vi "ZLIB Write File__ogtk.vi"(5 "error in (no error)":errorcluster, 7 "source path":path, 8 "zip Refnum":T1) -> (0 "error out":errorcluster, 3 "zip Refnum out":T1)   [LabVIEW 2014]
doc: "Writes a file from disk into the ZIP archive at the currently created file entry."
uses:
  <userlib>/_OpenG.lib/lvzip/lvzip.llb/ZLIB Zip Handle__ogtk.ctl
  <userlib>/_OpenG.lib/lvzip/lvzlib.dll
panel:
  # "Please visit http://www.OpenG.org to learn about the\nOpen Source LabVIEW software movement.\n\nNOTICE -- YOU MUST LEAVE THIS NOTICE IN PLACE.  PER THE TERMS OF THE LICENSE BELOW, YOU MAY SUBLICENSE THIS SOFTWARE \nIN ANY WAY THAT DOES NOT CONFLICT WITH THIS LICENSE.\n\n### BSD License (http://www.opensource.org/licenses/bsd-license.php) Begin ###\n \nCopyright (C) 2002-2004 Rolf Kalbermatter rolf.kalbermatter@citeng.com\nCopyright (C) 2002 Jim Kring jim@jimkring.com\n\nAll rights reserved.\n\nRedistribution and use in source and binary forms, with or without modification, are permitted provided that the following conditions are met:\n\n    * Redistributions of source code must retain the above copyright notice, this list of conditions and the following disclaimer.\n    * Redistributions in binary form must reproduce the above copyright notice, this list of conditions and the following disclaimer in the \n       documentation and/or other materials provided with the distribution.\n    * Neither the name of SciWare, James Kring, Inc., nor the names of its contributors may be used to endorse or promote products derived \n       from this software without specific prior written permission.\n\nTHIS SOFTWARE IS PROVIDED BY THE COPYRIGHT HOLDERS AND CONTRIBUTORS \"AS IS\" AND ANY EXPRESS OR IMPLIED WARRANTIES, \nINCLUDING, BUT NOT LIMITED TO, THE IMPLIED WARRANTIES OF MERCHANTABILITY AND FITNESS FOR A PARTICULAR PURPOSE ARE \nDISCLAIMED. IN NO EVENT SHALL THE COPYRIGHT OWNER OR CONTRIBUTORS BE LIABLE FOR ANY DIRECT, INDIRECT, INCIDENTAL,\n SPECIAL, EXEMPLARY, OR CONSEQUENTIAL DAMAGES (INCLUDING, BUT NOT LIMITED TO, PROCUREMENT OF SUBSTITUTE GOODS OR \nSERVICES; LOSS OF USE, DATA, OR PROFITS; OR BUSINESS INTERRUPTION) HOWEVER CAUSED AND ON ANY THEORY OF LIABILITY, \nWHETHER IN CONTRACT, STRICT LIABILITY, OR TORT (INCLUDING NEGLIGENCE OR OTHERWISE) ARISING IN ANY WAY OUT OF THE USE \nOF THIS SOFTWARE, EVEN IF ADVISED OF THE POSSIBILITY OF SUCH DAMAGE.\n\n### BSD License End ###"
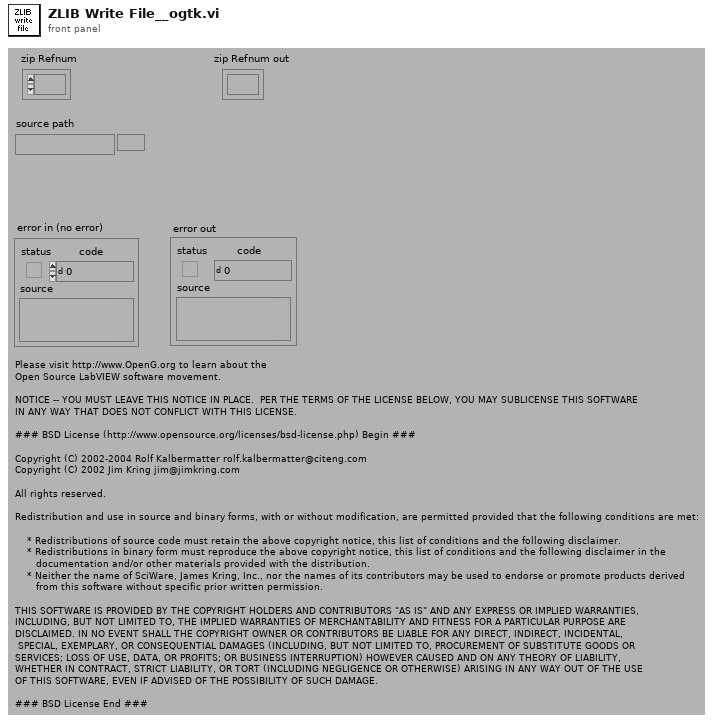
[diagram p1: front panel]
types:
  T1 = typedef "ZLIB Zip Handle__ogtk.ctl" = refnum<k1>
  T2 = enum16{"deny read/write", "deny write-only", "deny none"}
  T3 = enum16{"read/write", "read-only", "write-only", "write-only (truncate)"}
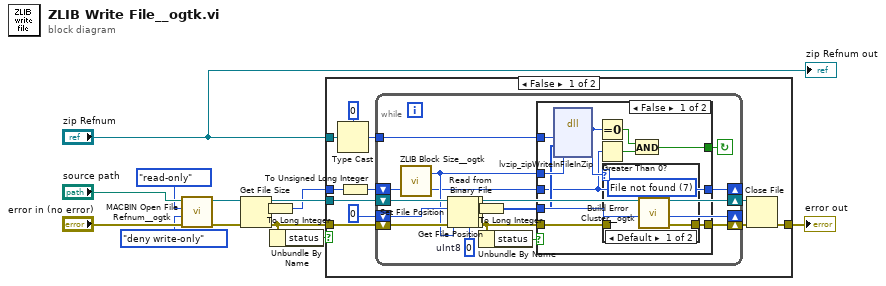
[diagram p0: block diagram]
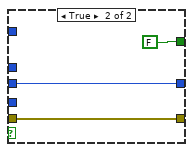
[diagram p3: hidden frame]
diagram:
  n1 = call <userlib>:"MACBIN Open File Refnum__ogtk.vi"("error in (no error)"="error in (no error)", "deny mode (2)"=T2."deny write-only", "open mode (0)"=T3."read-only", "file path"="source path") -> ("error out"=w6:errorcluster, "file refnum"=w5:refnum<file>)  [unwired: 3 in]
  n2 = Get File Size(file=w5, error in=w6) -> (refnum out=w3:refnum<file>, size (in bytes)=w1:i64, 0:w4:errorcluster)
  n3 = To Long Integer(number=w1) -> (32bit integer=w2:i32)
  n4 = Unbundle By Name(w4) -> ("status"=w12:bool)
  n5 = case shown="False" w12 {
    tunnel: w4 -> [w20 w61]
    tunnel: [w16 w61] -> w13
    tunnel: "zip Refnum" -> [w23 _]
    tunnel: w3 -> [w21 _]
    tunnel: w2 -> [w15 _]
    frame False {
      n6 = Type Cast(type=u32 0 ("unzFile"), x=w23) -> (*(type *) &x=w24:u32)
      n7 = To Unsigned Long Integer(number=w15) -> (unsigned 32bit integer=w14:u32)
      n8 = while {
        shift-left: w14 -> [w33]
        shift-right: [w30] -> _
        shift-left: w21 -> [w38]
        shift-right: [w38] -> w18
        shift-left: w20 -> [w42]
        shift-right: [w43] -> w17
        shift-left: 0 ("offset") -> [w41]
        shift-right: [w37] -> _
        tunnel: w24 -> [w44]
        stop <- w35 continue-if-true
        w40 = u8 0  # uInt8
        n9 = call <userlib>:"ZLIB Block Size__ogtk.vi"("length in"=w33) -> ("length rem"=w31:u32, "block len"=w32:u32)  [unwired: 1 in]
        n10 = Set File Position(offset (in bytes) (0)=w41, refnum=w38, error in=w42) -> (refnum out=w29:refnum<file>, error out=w28:errorcluster)  [unwired: 1 in]
        n11 = Read from Binary File(5:w40, 8:w28, 10:w32, 11:w29) -> (0:w26:errorcluster, 2:w39:u8[], 3:w27:refnum<file>)  [unwired: 2 in, 1 out]
        n12 = Get File Position(4:w26, 7:w27) -> (0:w36:errorcluster, 2:w25:i64)  [unwired: 1 out]
        n13 = To Long Integer(number=w25) -> (32bit integer=w37:i32)
        n14 = Unbundle By Name(w36) -> ("status"=w34:bool)
        n15 = case shown="False" w34 {
          tunnel: w44 -> [w54 _]
          tunnel: w32 -> [w53 _]
          tunnel: [w51 w59] -> w43
          tunnel: w39 -> [w50 _]
          tunnel: w36 -> [w49 w59]
          tunnel: [w46 FALSE] -> w35
          tunnel: w31 -> [w45 w58]
          tunnel: [w45 w58] -> w30
          frame False {
            n16 = dll-call lib="C:/Program Files (x86)/National Instruments/LabVIEW 2014/user.lib/_OpenG.lib/lvzip/lvzlib.*" fn="lvzip_zipWriteInFileInZip"("unzFile"=w54, "buffer"=w50, "size"=w53) -> (w52:i32)  [unwired: 6 in, 2 out]
            n17 = Equal To 0?(x=w52) -> (x = 0?=w48:bool)
            n18 = Greater Than 0?(x=w45) -> (x > 0?=w47:bool)
            n19 = case shown="Default" w52 {
              tunnel: w49 -> [_ w57]
              tunnel: [w56 w57] -> w51
              frame Default {
                w55 = 7 items=["No error", "Argument error", "Memory is full", "Out of zone", "End of file", "File already open", "Generic file I/O error", "File not found", "File permission error", "Disk is full", "Duplicate path", "Too many files open", "System feature not enabled", "Resource file not found", "Cannot add resource", "Resource not found", "Image not found", "Image memory error", "Pen does not exist", "Config type invalid", "Config token not found", "Config parse error", "Config memory error", "Bad external code format", "Bad external code offset", "External code not present", "Null window", "Destroy window error", "Null menu", "Print aborted", "Bad print record", "Print driver error", "Windows error during printing", "Memory error during printing", "Print dialog error", "Generic print error", "Invalid device refnum", "Device not found", "Device parameter error", "Device unit error", "Cannot open device", "Device call aborted", "Generic error", "Cancelled by user", "Object ID too low", "Object ID too high", "Object not in heap", "Unknown heap", "Unknown object (invalid DefProc)", "Unknown object (DefProc not in table)", "Message out of range", "Invalid (null) method", "Unknown message", "Manager call not supported", "Bad address", "Network operation in progress", "Network operation timed out", "Connection is busy", "Network attribute not supported", "Network error", "Address in use", "System out of memory", "Connection aborted", "Connection refused", "Not connected", "Already connected", "Connection closed", "Initialization error (interapplication manager)", "Bad occurrence", "Wait on unbound occurrence handler", "Occurrence queue overflow", "Datalog type conflict", "Unused", "Unrecognized type (interapplication manager)", "Memory corrupt", "Failed to make temporary DLL", "Old CIN version", "Drag socket not found", "Failed to load drop-object", "Failed to register OLE object", "Failed to release OLE object", "Format specifier type mismatch", "Unknown format specifier", "Too few format specifiers", "Too many format specifiers", "Scan failed", "Newer CIN version", "Error converting to variant", "Runtime menu error", "Password tampered", "Variant attribute not found", "Incompatible variant data type", "Event data is not available", "Event Store is not present", "Occurrence is not found", "Event Queue is not created", "Event info is not available", "Refnum passed is NULL", "Error retrieving Class GUID", "Error retrieving CoClass GUID", "Error retrieving TypeLib GUID.", "Bad built application magic bytes.", "Specific driver is different from the specific driver associated with the Logical Name.", "There is no session opened to the class driver.", "Max Error", "MAX - Error with config objects", "MAX - Error loading configuration", "MAX - Group not supported"]
                n20 = call <userlib>:"Build Error Cluster__ogtk.vi"("code"=w55) -> ("error out"=w56:errorcluster)  [unwired: 1 in]
              }
              frame 0 {
              }
            }
            n21 = And(x=w48, y=w47) -> (x .and. y?=w46:bool)
          }
          frame True {
          }
        }
      }
      n22 = Close File(refnum=w18, error in=w17) -> (error out=w16:errorcluster)  [unwired: 1 out]
    }
    frame True {
    }
  }
  "error out" <- w13
  "zip Refnum out" <- "zip Refnum"
